vi "test_alignLeftWithValidation.vi"(11 "Test Case In":refnum<class "RelativeAlignmentTests.lvclass">) -> (0 "error out":errorcluster, 3 "Test Case Out":refnum<class "RelativeAlignmentTests.lvclass">)   [LabVIEW 2023, in "RelativeAlignmentTests.lvclass"]
uses:
  RelativeAlignmentTests.lvclass
  C:/Program Files (x86)/National Instruments/LabVIEW 2023/vi.lib/Astemes/LUnit/Test Case.lvclass
  <vilib>/Astemes/LUnit/Test Case.lvclass/Test Case.ctl
  <vilib>/Astemes/LUnit/Core/LUnit Test Case/Private/Append Fail Result.vi
  <vilib>/Astemes/LUnit/Core/LUnit Test Case/Private/Append Pass Result.vi
  <vilib>/Astemes/LUnit/Core/LUnit Test Case/Private/Run In UI.vi
  <vilib>/Utility/error.llb/Clear Errors.vi
  RelativeAlignmentTests.lvclass/RelativeAlignmentTests.ctl
  <vilib>/Astemes/LUnit/Test Case.lvclass
  source/TLC_Geometry.lvlib
  C:/Program Files (x86)/National Instruments/LabVIEW 2023/vi.lib/Astemes/LUnit/LUnit Runnable.lvclass
  C:/projects/TLC_Geometry/tests/RelativeAlignmentTests/RelativeAlignmentTests.lvclass
panel:
  in  "movingObject":string
  in  "anchor":dbl
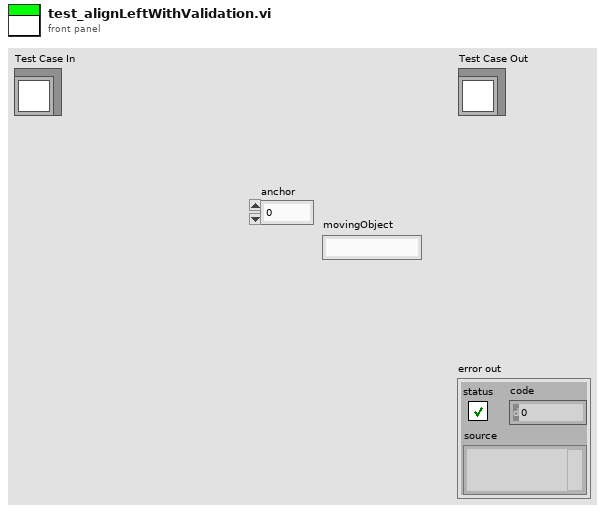
[diagram p1: front panel]
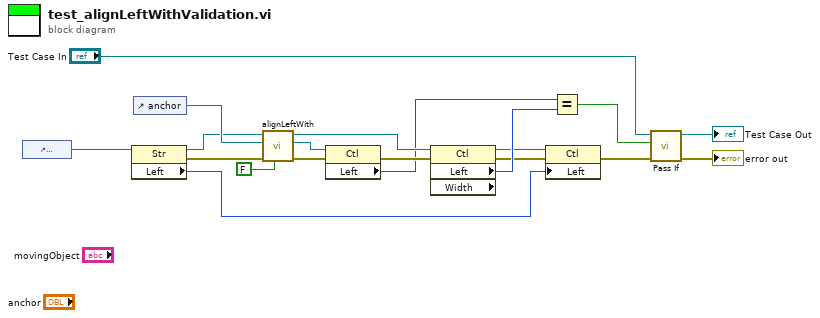
[diagram p0: block diagram]
diagram:
  n1 = control-ref of="movingObject"() -> (w9:refnum<vi>)
  n2 = property class="Str"(reference=w9) -> (reference out=w8:refnum<vi>, error out=w17:errorcluster, "Left"=w5:i32)  [unwired: 1 in]
  n3 = control-ref of="anchor"() -> (w18:refnum<vi>)
  n4 = call "alignLeftWith.vi"("useControlBodyOnly"=FALSE, "error in (no error)"=w17, "anchorObject"=w18, "movingObject"=w8) -> ("error out"=w15:errorcluster, "anchorObject(dup)"=w13:refnum<vi>, "movingObject(dup)"=w12:refnum<vi>)  [unwired: 5 in]
  n5 = property class="Ctl"(reference=w13, error in=w15) -> (error out=w14:errorcluster, "Left"=w7:i32)  [unwired: 1 out]
  n6 = property class="Ctl" props=["Left", "Width"](reference=w12, error in=w14) -> (reference out=w10:refnum<vi>, error out=w11:errorcluster, "Left"=w16:i32)  [unwired: 1 out]
  n7 = property class="Ctl"(reference=w10, error in=w11, "Left"=w5) -> (error out=w6:errorcluster)  [unwired: 1 out]
  n8 = Equal?(x=w7, y=w16) -> (x = y?=w4:bool)
  n9 = call <vilib>:"Pass If.vi"("error in (no error)"=w6, "Pass?"=w4, "LUnit Test Case In"="Test Case In") -> ("error out"=→"error out":errorcluster, "LUnit Test Case Out"=→"Test Case Out":refnum<class "RelativeAlignmentTests.lvclass">)  [unwired: 7 in]
